vi "RT Driver VI.vi"(7 "Operation":T1, 11 "Device Reference in":T2 format="%.0x") -> (0 "Error Code":i32)   [LabVIEW 2019, in "HLA Custom Device Engine.lvlib"]
uses:
  HLA Custom Device Engine.lvlib
  <vilib>/NI VeriStand/Custom Device API/Custom Device Item Ref.ctl
  <vilib>/NI VeriStand/Custom Device API/Hardware Interface Driver VI Operation.ctl
  <vilib>/NI/NIVS Inline Async API/_VS Inline Async API/VS Inline Async API/VS Inline Async API.lvclass
  <vilib>/NI/NIVS Inline Async API/_VS Inline Async API/VS Inline Async API/VS Inline Async API.lvclass/VS Inline Async API.ctl
  <vilib>/NI/NIVS Inline Async API/_Data Access Engine/Data Access Engine/Data Access Engine.lvclass/Data Access Engine.ctl
  <vilib>/NI/NIVS Inline Async API/_Data Access Engine/Access Type Classes/Write/Write.lvclass/Write.ctl
  <vilib>/NI/NIVS Inline Async API/_Data Access Engine/Access Type Classes/ReadWrite/ReadWrite.lvclass/ReadWrite.ctl
  <vilib>/NI/NIVS Inline Async API/_Data Access Engine/Access Type Classes/Read/Read.lvclass/Read.ctl
  <vilib>/NI/NIVS Inline Async API/_Data Access Engine/Data Access Engine/Methods/Data.Engine.Read Data from HW.vi
  <vilib>/NI/NIVS Inline Async API/_VS Inline Async API/Error Handling Process/SubVIs/Error.GetError.vi
  <vilib>/NI/NIVS Inline Async API/_Data Access Engine/Data Access Engine/Methods/Data.Engine.Write Data to HW.vi
  <vilib>/NI/NIVS Inline Async API/_Data Access Engine/Access Type Classes/ReadWrite/ReadWrite.EngineData.vi
  <vilib>/NI/NIVS Inline Async API/_Data Access Engine/Access Type Classes/Write/Write.EngineData.vi
  <vilib>/NI/NIVS Inline Async API/_Data Access Engine/Access Type Classes/Read/Read.EngineData.vi
  <vilib>/NI VeriStand/Custom Device API/NI VeriStand - Get Channel Value by Data Reference.vi
  <vilib>/NI VeriStand/Custom Device API/NI VeriStand - Set Channel Value by Data Reference.vi
  <vilib>/NI VeriStand/Custom Device API/NI VeriStand - Get Channel Values by Block Data Reference.vi
  Shared/Constants.vi
  <vilib>/NI VeriStand/Custom Device API/Global Data Refs.vi
  <vilib>/NI VeriStand/Custom Device API/Get Item Property (Variant).vi
  <vilib>/NI VeriStand/Custom Device API/Custom Device API.lvlib
  <vilib>/NI VeriStand/Custom Device Tools/Custom Device Utility Library/Custom Device Utility Library.lvlib
  Shared/Compiled.Settings.ctl
  Shared/HLA Custom Device Shared.lvlib
  RTStateVariables.ctl
  RTinlineRuntimeData.ctl
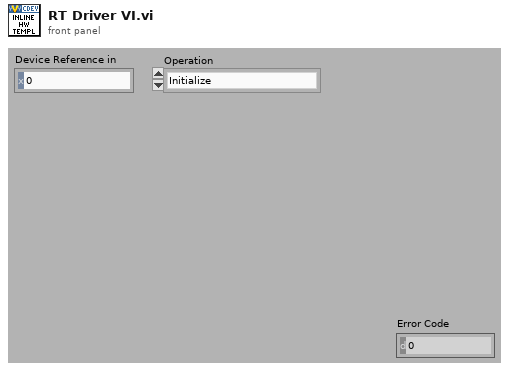
[diagram p1: front panel]
types:
  T1 = typedef "Custom Device API.lvlib/Hardware Interface Driver VI Operation.ctl" = enum16{"Initialize", "Start", "Read Data from HW", "Write Data to HW", "Close"}
  T2 = typedef "Custom Device API.lvlib/Custom Device Item Ref.ctl" = u64
  T3 = typedef "HLA Custom Device Engine.lvlib/RTStateVariables.ctl" = cluster{"Async":refnum<class "VS Inline Async API.lvclass">, "Settings":T4, "inline runtime data":T5}
  T4 = typedef "HLA Custom Device Shared.lvlib/Compiled.Settings.ctl" = cluster{"Name":string, "Async Init Timeout":u16}
  T5 = typedef "HLA Custom Device Engine.lvlib/RTinlineRuntimeData.ctl" = cluster{"Numeric":dbl}
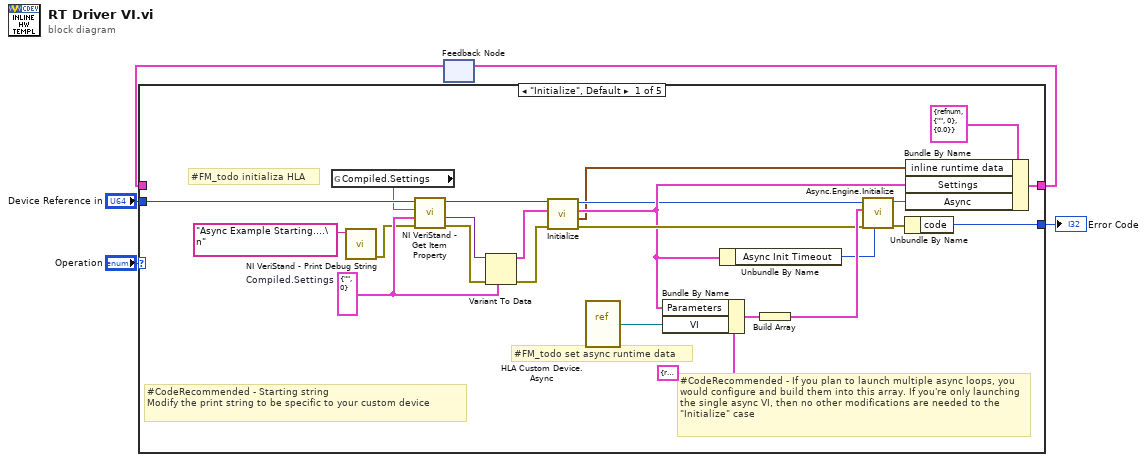
[diagram p0: block diagram]
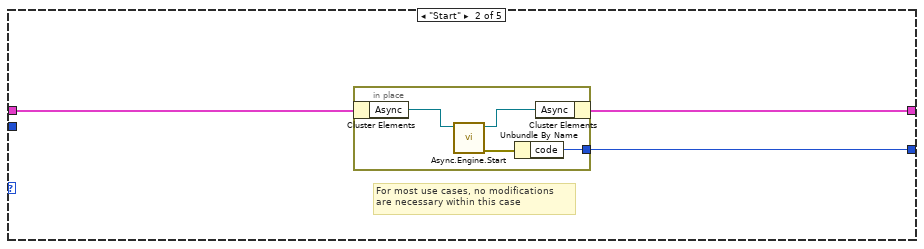
[diagram p2: hidden frame]
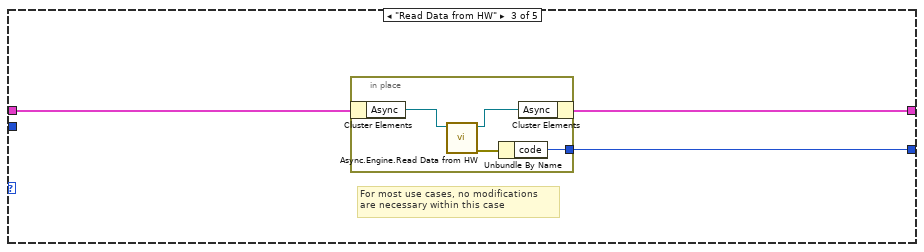
[diagram p3: hidden frame]
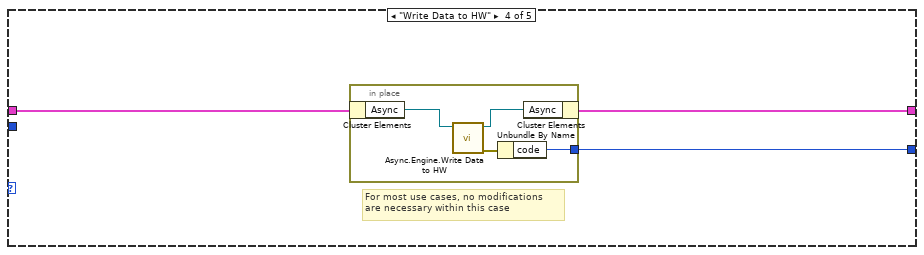
[diagram p4: hidden frame]
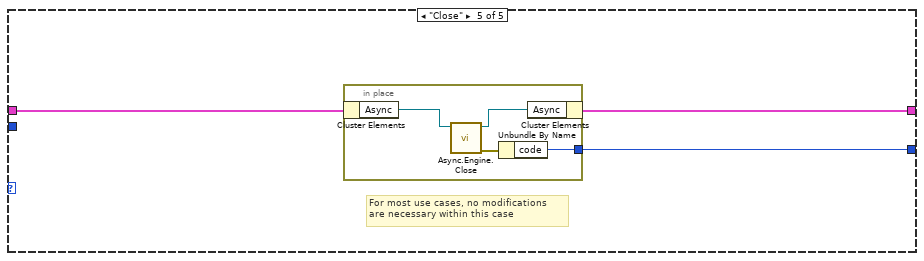
[diagram p5: hidden frame]
diagram:
  n1 = feedback #1() -> (w3:T3)  [unwired: 1 out]
  n2 = case shown="\"Initialize\", Default" "Operation" {
    tunnel: [w27 w31 w37 w44 w52] -> w4
    tunnel: w3 -> [_ w32 w39 w45 w53]
    tunnel: "Device Reference in" -> [w24 _ _ _ _]
    tunnel: [w29 w30 w38 w46 w51] -> w1
    frame "Initialize", Default {
      w19 = T4 {"Name"="", "Async Init Timeout"=0}  # Compiled.Settings
      # "#FM_todo set async runtime data"
      # "#FM_todo initializa HLA"
      # "#CodeRecommended - Starting string\nModify the print string to be specific to your custom device"
      # "#CodeRecommended - If you plan to launch multiple async loops, you would configure and build them into this array. If you're only launching the single async VI, then no other modifications are needed to the \"Initialize\" case"
      n3 = global read "Constants.vi" "Compiled.Settings"() -> (w21:string)
      n4 = call <vilib>:"NI VeriStand - Print Debug String.vi"("Message"="Async Example Starting....\n") -> ("error out"=w17:errorcluster)  [unwired: 10 in]
      n5 = call-poly <vilib>:"NI VeriStand - Get Item Property.vi"("error in (no error)"=w17, "Default Value"=w19, "Property Name"=w21, "Item Ref in"=w24) -> ("error out"=w23:errorcluster, "Value"=w22:variant, "Item Ref out"=w13:T2)  [unwired: 4 in, 1 out]
      n6 = Variant To Data(error in=w23, type=w19, Variant=w22) -> (data=w10:T4, error out=w12:errorcluster)
      n7 = call "Initialize.vi"("error in"=w12, "settings in"=w10, "Device Reference in"=w13) -> ("error out"=w11:errorcluster, "inline runtime data"=w6:T5, "settings out"=w9:T4, "Device Reference out"=w8:T2)  [unwired: 5 in]
      n8 = vi-ref "HLA Custom Device.Async.vi"() -> (w15:refnum<vi>)
      n9 = Bundle By Name(cluster=cluster{"VI":refnum<vi>, "Parameters":variant} {"VI"=refnum, "Parameters"=variant} ("Process"), "Parameters"=w9, "VI"=w15) -> (w25:cluster{"VI":refnum<vi>, "Parameters":variant})
      n10 = Unbundle By Name(w9) -> ("Async Init Timeout"=w14:u16)
      n11 = Build Array(w25) -> (w18:cluster{"VI":refnum<vi>, "Parameters":variant}[])
      n12 = call <vilib>:"Async.Engine.Initialize.vi"("Timeout (ms) (5000)"=w14, "error in (no error)"=w11, "Processes"=w18, "Custom Device Ref"=w8) -> ("error out"=w20:errorcluster, "Async"=w28:refnum<class "VS Inline Async API.lvclass">)  [unwired: 6 in]
      n13 = Unbundle By Name(w20) -> ("code"=w29:i32)
      n14 = Bundle By Name(cluster=T3 {"Async"=refnum, "Settings"={"Name"="", "Async Init Timeout"=0}, "inline runtime data"={"Numeric"=0.0}} ("RT State Variables"), "inline runtime data"=w6, "Settings"=w9, "Async"=w28) -> (w27:T3)
    }
    frame "Start" {
      # "For most use cases, no modifications \nare necessary within this case"
      n15 = in-place {
        in-place-border: [w33] -> w30
        n16 = in-place-cluster #2(w32) -> ("Async"=w36:refnum<class "VS Inline Async API.lvclass">)
        n17 = call <vilib>:"Async.Engine.Start.vi"("VS Inline Async API in"=w36) -> ("error out"=w34:errorcluster, "VS Inline Async API out"=w35:refnum<class "VS Inline Async API.lvclass">)  [unwired: 9 in]
        n18 = Unbundle By Name(w34) -> ("code"=w33:i32)
        n19 = in-place-cluster #2("Async"=w35) -> (w31:T3)
      }
    }
    frame "Read Data from HW" {
      # "For most use cases, no modifications \nare necessary within this case"
      n20 = in-place {
        in-place-border: [w41] -> w38
        n21 = in-place-cluster #3(w39) -> ("Async"=w43:refnum<class "VS Inline Async API.lvclass">)
        n22 = call <vilib>:"Async.Engine.Read Data from HW.vi"("Async in"=w43) -> ("error out"=w40:errorcluster, "Async out"=w42:refnum<class "VS Inline Async API.lvclass">)  [unwired: 9 in]
        n23 = Unbundle By Name(w40) -> ("code"=w41:i32)
        n24 = in-place-cluster #3("Async"=w42) -> (w37:T3)
      }
    }
    frame "Write Data to HW" {
      # "For most use cases, no modifications \nare necessary within this case"
      n25 = in-place {
        in-place-border: [w50] -> w46
        n26 = in-place-cluster #4(w45) -> ("Async"=w48:refnum<class "VS Inline Async API.lvclass">)
        n27 = call <vilib>:"Async.Engine.Write Data to HW.vi"("VS Inline Async API in"=w48) -> ("error out"=w49:errorcluster, "VS Inline Async API out"=w47:refnum<class "VS Inline Async API.lvclass">)  [unwired: 9 in]
        n28 = Unbundle By Name(w49) -> ("code"=w50:i32)
        n29 = in-place-cluster #4("Async"=w47) -> (w44:T3)
      }
    }
    frame "Close" {
      # "For most use cases, no modifications \nare necessary within this case"
      n30 = in-place {
        in-place-border: [w55] -> w51
        n31 = in-place-cluster #5(w53) -> ("Async"=w57:refnum<class "VS Inline Async API.lvclass">)
        n32 = call <vilib>:"Async.Engine.Close.vi"("Async in"=w57) -> ("error out"=w54:errorcluster, "Async out"=w56:refnum<class "VS Inline Async API.lvclass">)  [unwired: 9 in]
        n33 = Unbundle By Name(w54) -> ("code"=w55:i32)
        n34 = in-place-cluster #5("Async"=w56) -> (w52:T3)
      }
    }
  }
  "Error Code" <- w1
  n35 = feedback-in #1(w4) -> ()
